vi "Detect Tags.vi"(7 "Region Offset (Default: 0,0)":T2, 8 "error in (no error)":errorcluster, 9 "Region Size (Default:0,0 - Whole Image)":T1, 10 "Greyscale Image in":T6, 11 "Apriltag Detector in":refnum<class "AprilTag Detector.lvclass">) -> (0 "error out":errorcluster, 1 "Computed Region Size":T1, 2 "Detections":T3[](array[typedef]), 3 "Apriltag Detector":refnum<class "AprilTag Detector.lvclass">, 4 "# Detections":i32)   [LabVIEW 2020, in "feature_detection.lvlib" / "AprilTag Detector.lvclass"]
doc: "Detect the Tags in the Greyscale Image."
uses:
  AprilTag Detector.lvclass
  image/Greyscale Image.ctl
  Detection.ctl
  common/Image Point (Float).ctl
  common/Quad Corners.ctl
  common/Image Point (Integer).ctl
  common/Image Size (Integer).ctl
  AprilTag Detector.lvclass/AprilTag Detector.ctl
  common/common.lvlib
  common/bin/gartoolkit_fd_32-1.dll
  image/image.lvlib
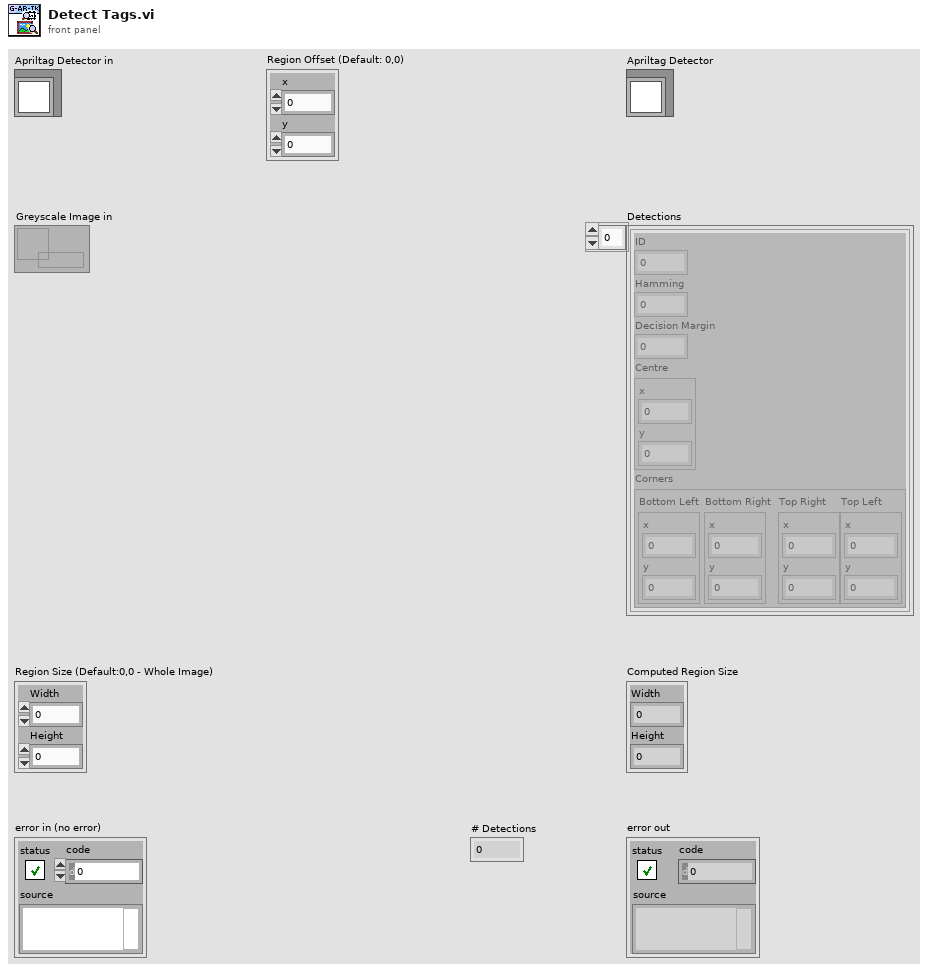
[diagram p1: front panel]
types:
  T1 = typedef "common.lvlib/Image Size (Integer).ctl" = cluster{"Width":u16, "Height":u16}
  T2 = typedef "common.lvlib/Image Point (Integer).ctl" = cluster{"x":i32, "y":i32}
  T3 = typedef "feature_detection.lvlib/AprilTag Detector.lvclass/Detection.ctl" = cluster{"ID":i32, "Hamming":i32, "Decision Margin":sgl, "Centre":T4, "Corners":T5}
  T4 = typedef "common.lvlib/Image Point (Float).ctl" = cluster{"x":dbl, "y":dbl}
  T5 = typedef "common.lvlib/Quad Corners.ctl" = cluster{"Bottom Left":T4, "Bottom Right":T4, "Top Right":T4, "Top Left":T4}
  T6 = typedef "image.lvlib/Greyscale Image.ctl" = refnum<data-value>
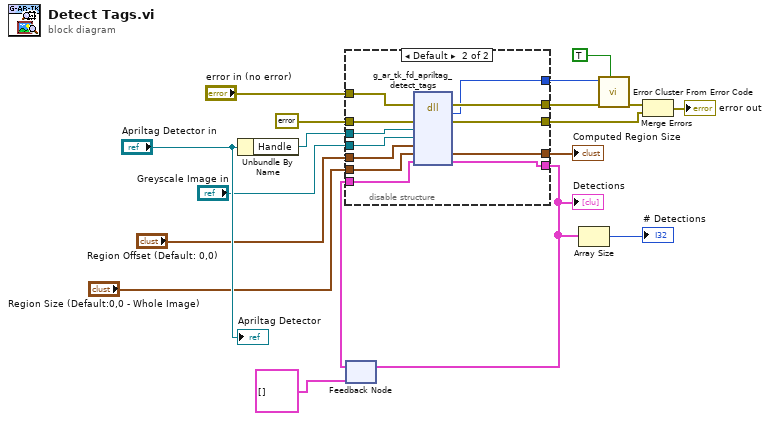
[diagram p0: block diagram]
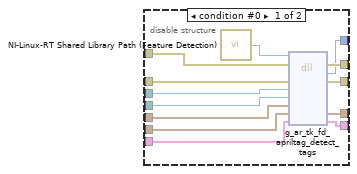
[diagram p2: hidden frame]
diagram:
  n1 = Unbundle By Name("Apriltag Detector in") -> ("Handle"=w12:refnum<data-value>)
  n2 = feedback #1(T3[] [] ("Array")) -> (w6:T3[])
  n3 = disable-structure shown="Default" {
    disable-tunnel: "error in (no error)" -> [w30 w43]
    disable-tunnel: errorcluster {"status"=FALSE, "code"=0, "source"=""} ("error constant") -> [w29 w42]
    disable-tunnel: w12 -> [w28 w41]
    disable-tunnel: "Greyscale Image in" -> [w27 w40]
    disable-tunnel: w6 -> [w26 w39]
    disable-tunnel: [w25 w38] -> w10
    disable-tunnel: [w24 w37] -> w9
    disable-tunnel: [w23 w36] -> w8
    disable-tunnel: [w22 w35] -> w7
    disable-tunnel: "Region Offset (Default: 0,0)" -> [w21 w34]
    disable-tunnel: "Region Size (Default:0,0 - Whole Image)" -> [w20 w33]
    disable-tunnel: [w19 w32] -> w1
    frame condition #0 {
      n4 = call "NI-Linux-RT Shared Library Path (Feature Detection).vi"() -> ("Path"=w31:path)
      n5 = dll-call lib="?" fn="g_ar_tk_fd_apriltag_detect_tags" ("g_ar_toolkit.*.*:g_ar_tk_capture_context_create")(path in=w31, error in=w30, "error_cluster"=w29, "Detector_EDVR"=w28, "Image_EDVR"=w27, "offset"=w21, "size"=w20, "Detections"=w26) -> (error out=w25:errorcluster, "return type"=w24:i32, "error_cluster"=w23:errorcluster, "size"=w19:T1, "Detections"=w22:T3[])  [unwired: 4 in, 1 out]
    }
    frame condition #1 (active) {
      n6 = dll-call lib="C:/serenial/lib/g-augmented-reality-toolkit/LabVIEW/common/bin/gartoolkit_fd_*-1.*" fn="g_ar_tk_fd_apriltag_detect_tags" ("g_ar_toolkit.*.*:g_ar_tk_capture_context_create")(error in=w43, "error_cluster"=w42, "Detector_EDVR"=w41, "Image_EDVR"=w40, "offset"=w34, "size"=w33, "Detections"=w39) -> (error out=w38:errorcluster, "return type"=w37:i32, "error_cluster"=w36:errorcluster, "size"=w32:T1, "Detections"=w35:T3[])  [unwired: 5 in, 1 out]
    }
  }
  "Detections" <- w7
  "Computed Region Size" <- w1
  n7 = feedback-in #1(w7) -> ()
  n8 = Array Size(array=w7) -> (size(s)=→"# Detections":i32)
  n9 = call <vilib>:"Error Cluster From Error Code.vi"("show call chain? (False)"=TRUE, "error in (no error)"=w10, "error code (0)"=w9) -> ("error out"=w17:errorcluster)  [unwired: 6 in]
  n10 = Merge Errors(w17, w8) -> (→"error out":errorcluster)
  "Apriltag Detector" <- "Apriltag Detector in"
